vi "Initialize.vi"(8 "error in (no error)":errorcluster, 11 "SAM in":refnum<class "SAM.lvclass">) -> (0 "error out":errorcluster, 3 "SAM out":refnum<class "SAM.lvclass">)   [LabVIEW 2020, in "SAM.lvclass"]
uses:
  SAM.lvclass
  D:/Experiment VIs/Signal Synthesis VIs/4th Generation/Classes/Modulations/AM/AM.lvclass
  SAM.lvclass/SAM.ctl
  AM/AM.lvclass/AM.ctl
  AM/Write vref.vi
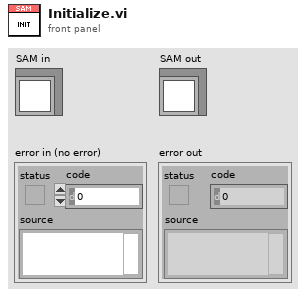
[diagram p1: front panel]
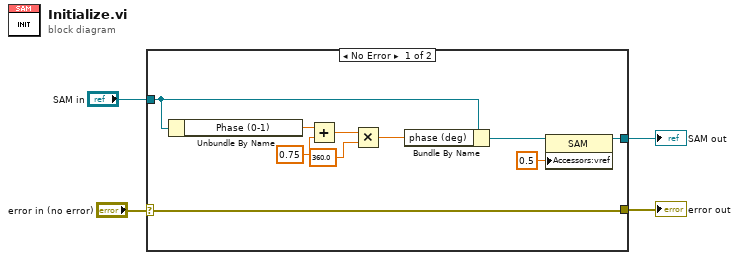
[diagram p0: block diagram]
diagram:
  n1 = case shown="No Error" "error in (no error)" {
    selector: "error in (no error)" -> [w8 w16]
    tunnel: [w8 w16] -> w2
    tunnel: "SAM in" -> [w7 w15]
    tunnel: [w6 w15] -> w1
    frame No Error {
      n2 = Unbundle By Name(w7) -> ("Phase (0-1)"=w12:dbl)
      n3 = Add(x=w12, y=0.75) -> (x+y=w14:dbl)
      n4 = Multiply(x=w14, y=360.0) -> (x*y=w10:dbl)
      n5 = Bundle By Name(cluster=w7, "phase (deg)"=w10) -> (w9:refnum<class "SAM.lvclass">)
      n6 = property class="SAM"(reference=w9, "Accessors:vref"=0.5 ("vref")) -> (reference out=w6:refnum<class "SAM.lvclass">)  [unwired: 1 in, 1 out]
    }
    frame Error {
    }
  }
  "error out" <- w2
  "SAM out" <- w1
